vi "serialRead.vi"(8 "error in (no error)":errorcluster, 11 "Python":T1) -> (0 "error out":errorcluster, 2 "Reply":string, 3 "Python out":T1)   [LabVIEW 2022 SP3]
uses:
  PythonCtrl.ctl
  Processors.ctl
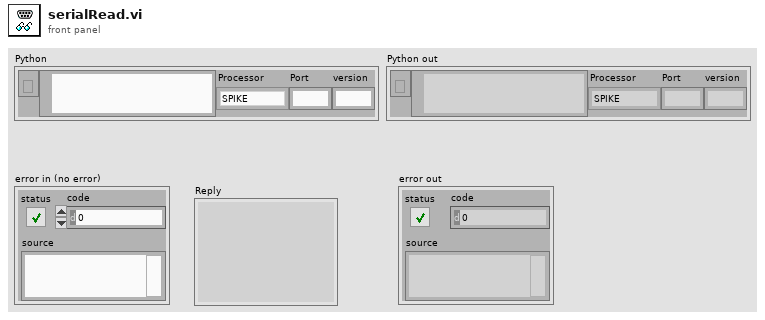
[diagram p1: front panel]
types:
  T1 = typedef "PythonCtrl.ctl" = cluster{"session":refnum<k35>, "PyPath":path, "Processor":T2, "Port":string, "version":string}
  T2 = typedef "Processors.ctl" = enum16{"SPIKE", "Pi", "Pi_ssh", "OpenMV", "Dunio"}
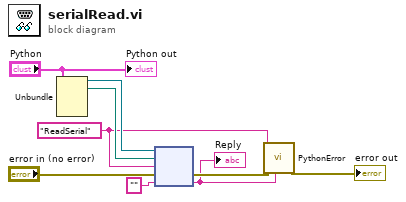
[diagram p0: block diagram]
diagram:
  w1 = "ReadSerial" ("function name")
  n1 = Unbundle("Python") -> ("session"=w8:refnum<k35>, "PyPath"=w9:path)  [unwired: 3 out]
  n2 = node(w8, w9, w1, "error in (no error)", "" ("function name")) -> (w4:errorcluster, w2:string)  [unwired: 3 out]
  "Reply" <- w2
  n3 = call "PythonError.vi"("reply"=w2, "error in (no error)"=w4, "function name"=w1) -> ("error out"=→"error out":errorcluster)  [unwired: 8 in]
  "Python out" <- "Python"
